vi "删除demo守护脚本文件.vi"(8 "错误输入":errorcluster) -> (0 "错误输出":errorcluster)   [LabVIEW 2016]
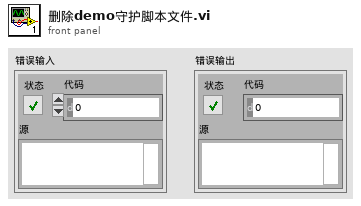
[diagram p1: front panel]
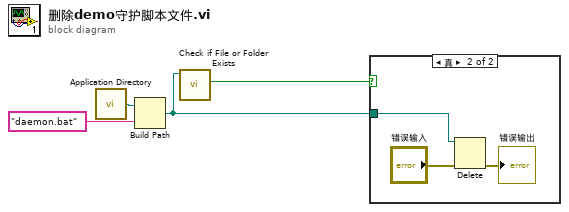
[diagram p0: block diagram]
diagram:
  n1 = call <vilib>:"Application Directory.vi"() -> ("Application Directory"=w3:path)
  n2 = Build Path(base path=w3, name or relative path="daemon.bat" ("字符串")) -> (appended path=w1:path)
  n3 = call <vilib>:"Check if File or Folder Exists.vi"("path"=w1) -> ("file or folder exists?"=w4:bool)  [unwired: 8 in, 2 out]
  n4 = case shown="真" w4 {
    tunnel: w1 -> [_ w5]
    frame False {
    }
    frame True {
      n5 = Delete(path (use dialog)=w5, error in="错误输入") -> (error out=→"错误输出":errorcluster)  [unwired: 3 in, 2 out]
    }
  }
